vi "Read Error .vi"(8 "error in (no error)":errorcluster, 11 "WebSocket Service Enqueuer Msg in":refnum<class "WebSocket Server-Service Enqueuer Msg.lvclass">) -> (0 "error out":errorcluster, 2 "Error":errorcluster, 3 "WebSocket Service Enqueuer Msg out":refnum<class "WebSocket Server-Service Enqueuer Msg.lvclass">)   [LabVIEW 2016, in "WebSocket Actors.lvlib" / "WebSocket Server-Service Enqueuer Msg.lvclass"]
uses:
  WebSocket Server-Service Enqueuer Msg.lvclass
  WebSocket Server-Service Enqueuer Msg.lvclass/WebSocket Server-Service Enqueuer Msg.ctl
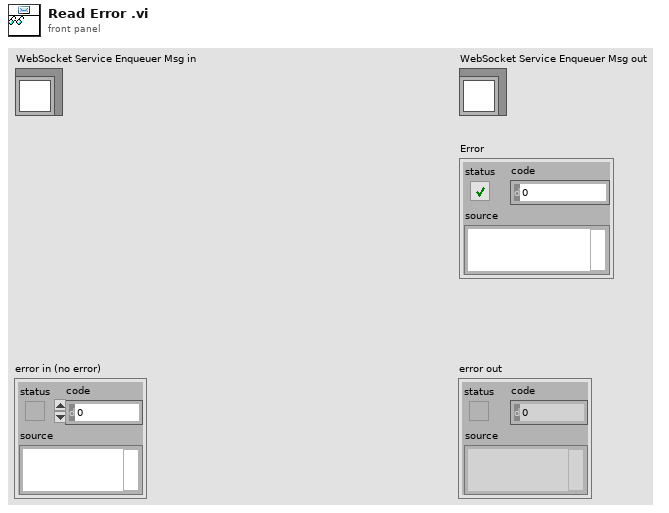
[diagram p1: front panel]
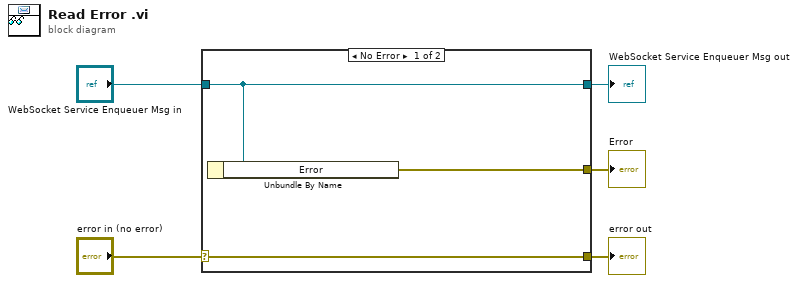
[diagram p0: block diagram]
diagram:
  n1 = case shown="No Error" "error in (no error)" {
    selector: "error in (no error)" -> [w8 w9]
    tunnel: [w8 w9] -> w4
    tunnel: [w7 w10] -> w2
    tunnel: "WebSocket Service Enqueuer Msg in" -> [w7 w10]
    tunnel: [w6 _] -> w1
    frame No Error {
      n2 = Unbundle By Name(w7) -> ("Error"=w6:errorcluster)
    }
    frame Error {
    }
  }
  "error out" <- w4
  "WebSocket Service Enqueuer Msg out" <- w2
  "Error" <- w1
